vi "Get DDGTTL Gate Width.vi"(8 "error in (no error)":errorcluster, 10 "ttlWidth":cluster{}, 11 "opticalWidth":cluster{}) -> (0 "error out":errorcluster, 2 "ttlWidth out":cluster{}, 3 "function return":u32)   [LabVIEW 2014, in "atmcd32d.lvlib"]
doc: "unsigned int WINAPI GetDDGTTLGateWidth(at_u64 opticalWidth, at_u64 * ttlWidth);"
uses:
  atmcd32d.lvlib
  atmcd32d.dll
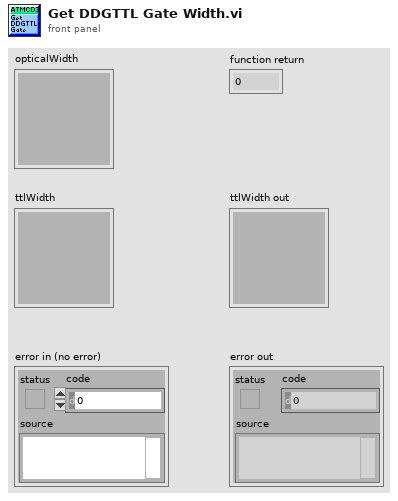
[diagram p1: front panel]
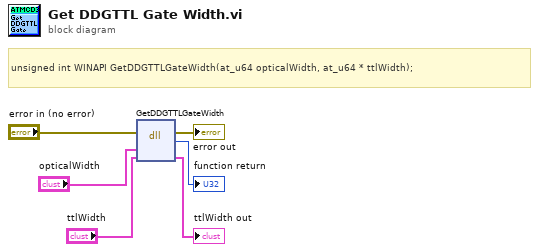
[diagram p0: block diagram]
diagram:
  # "unsigned int WINAPI GetDDGTTLGateWidth(at_u64 opticalWidth, at_u64 * ttlWidth);"
  n1 = dll-call lib="C:/Users/Bakir/Documents/Lambda2-Testing/lib/Andorlib/atmcd32d.*" fn="GetDDGTTLGateWidth"(error in="error in (no error)", "opticalWidth"="opticalWidth", "ttlWidth"="ttlWidth") -> (error out=→"error out":errorcluster, →"function return":u32, "ttlWidth"=→"ttlWidth out":cluster{})  [unwired: 3 in, 1 out]
